vi "macro_SngJntArm_Sim_Execute.vi"() -> ()   [LabVIEW 2019, in "Trajectory_Library.lvlib"]
uses:
  Trajectory_Library.lvlib
  Enum/DCMOTOR_TYPES_ENUM.ctl
  BatterySim_CalculateLoadedBatteryVoltage.vi
panel:
  in  "Motor Dmd (CO)":dbl
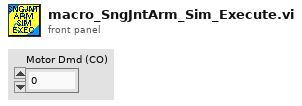
[diagram p1: front panel]
types:
  T1 = typedef "Trajectory_Library.lvlib/DCMOTOR_TYPES_ENUM.ctl" = enum16{"CIM", "AndyMark 9015", "Andy Mark RS 775 125", "Bag", "BaneBots RS 550", "BaneBots RS 775", "Falcon 500", "Mini CIM", "NEO", "NEO 550", "Romi BuiltIn", "Vex 775 Pro", "Snow Blower AM 2235A", "Bosch Seat AM 3493"}
  T2 = typedef "Trajectory_Library.lvlib/LINEAR_SYSTEM_ID_SINGLE_JOINT_ARM_MODEL.ctl" = cluster{"DCMOTOR_TYPES":T1, "Num Motors":i32, "ArmLength_M":dbl, "massKg":dbl, "Gearing":dbl, "MOI kgm2":dbl, "Estimate MOI":bool}
  T3 = typedef "Trajectory_Library.lvlib/SINGLE_JOINT_ARM_SIM_SIMULATION_PARAMS.ctl" = cluster{"MinAngle_Rad":dbl, "MaxAngle_Rad":dbl, "Measurment StdDev":dbl, "SimulateGravity":bool}
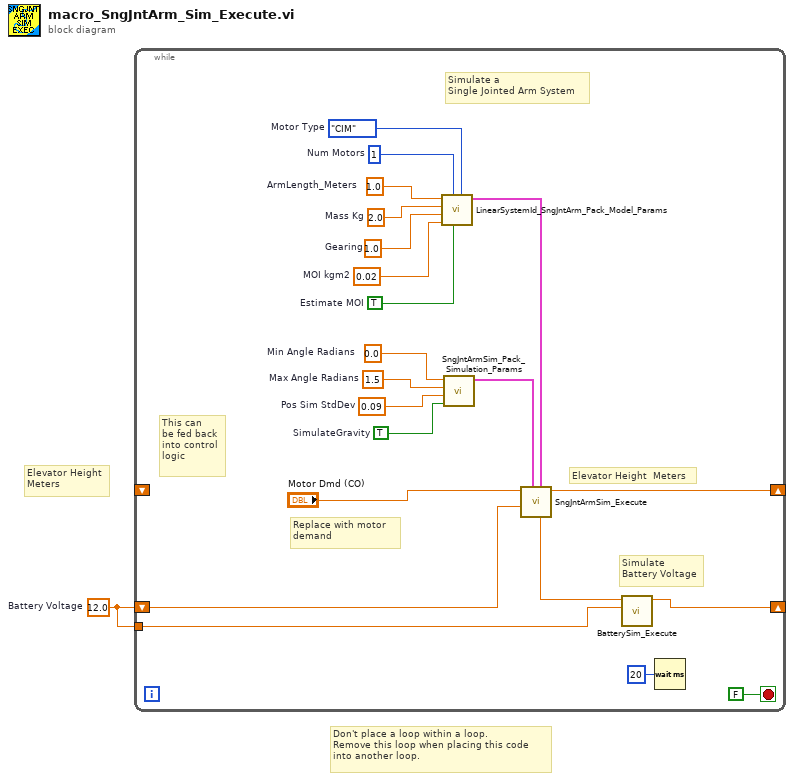
[diagram p0: block diagram]
diagram:
  w1 = 12.0  # Battery Voltage
  # "Don't place a loop within a loop. \nRemove this loop when placing this code\ninto another loop."
  # "Elevator Height\nMeters"
  n1 = while {
    shift-right: [w15] -> _
    shift-left: w1 -> [w13]
    shift-right: [w14] -> _
    shift-left: _ -> [_]
    tunnel: w1 -> [w2]
    stop <- FALSE stop-if-true
    w6 = TRUE  # Estimate MOI
    w7 = 0.02  # MOI kgm2
    w8 = 0.0  # Min Angle Radians
    w9 = 1.5  # Max Angle Radians
    w10 = 0.09  # Pos Sim StdDev
    w11 = TRUE  # SimulateGravity
    w12 = 1.0  # ArmLength_Meters
    w19 = 1.0  # Gearing
    w20 = 2.0  # Mass Kg
    w21 = 1  # Num Motors
    w22 = DCMOTOR_TYPES_ENUM."CIM"  # Motor Type
    # "This can\nbe fed back\ninto control\nlogic"
    # "Elevator Height  Meters"
    # "Replace with motor \ndemand"
    # "Simulate\nBattery Voltage"
    # "Simulate a\nSingle Jointed Arm System"
    n2 = call "LinearSystemId_SngJntArm_Pack_Model_Params.vi"("DCMOTOR_TYPES"=w22, "Estimate MOI"=w6, "Num Motors"=w21, "MOI kgm2"=w7, "Gearing"=w19, "massKg"=w20, "ArmLength_M"=w12) -> ("SngJntArmSim_Model _Params"=w5:T2)  [unwired: 4 in]
    n3 = call "SngJntArmSim_Pack_Simulation_Params.vi"("SimulateGravity"=w11, "Pos Sim StdDev Rad"=w10, "MaxAngle_Rad"=w9, "MinAngle_Rad"=w8) -> ("SngJntArmSim_Simulation _Params"=w4:T3)  [unwired: 7 in]
    n4 = call "SngJntArmSim_Execute.vi"("SngJntArmSim_Model _Params"=w5, "SngJntArmSim_Simulation _Params"=w4, "Battery Volts"=w13, "Motor Dmd"="Motor Dmd (CO)") -> ("ArmAngle_Rad"=w14:dbl, "Motor Current"=w16:dbl)  [unwired: 2 in, 4 out]
    n5 = call "BatterySim_Execute.vi"("Nominal Battery Voltage"=w2, "Current"=w16) -> ("Voltage"=w15:dbl)  [unwired: 9 in]
    n6 = Wait (ms)(milliseconds to wait=u32 20) -> ()  [unwired: 1 out]
  }
